vi "DBLToI64.vi"(5 "Number":dbl) -> (1 "Signed 64-bit integer":i64, 2 "Overflow?":bool, 3 "Exact conversion?":bool)   [LabVIEW 2017, in "GPOverflow.lvlib"]
doc: "Converts <B>Number</B> to I64 keeping track of numeric overflow and exactness of conversion.\n\n<B>Exact conversion?</B> will be True only if a conversion back into the original data type of <B>Number</B> will yield the exact same number, i.e. no precision was lost during the conversion.\n\n<B>Overflow?</B> will be True if positive or negative overflow occurred. The numeric output will saturate in case of overflow.\n\nThis VI is inlined.\n\nSteen Schmidt\nGPower\n6/3 2013"
uses:
  GPOverflow.lvlib
  Comparison/GPComparison.lvlib
  Comparison/Library/IsInt/IsIntDBL.vi
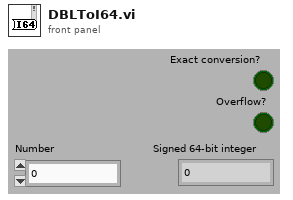
[diagram p1: front panel]
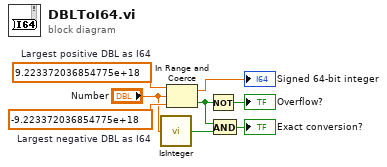
[diagram p0: block diagram]
diagram:
  w7 = -9.223372036854775e+18  # Largest negative DBL as I64
  w8 = 9.223372036854775e+18  # Largest positive DBL as I64
  n1 = call-poly "IsInteger.vi"("x"="Number") -> ("Integer?"=w2:bool)  [unwired: 4 in]
  n2 = In Range and Coerce(upper limit=w8, x="Number", lower limit=w7) -> (coerced(x)=→"Signed 64-bit integer":dbl, In Range?=w3:bool)
  n3 = Not(x=w3) -> (.not. x?=→"Overflow?":bool)
  n4 = And(x=w3, y=w2) -> (x .and. y?=→"Exact conversion?":bool)
